vi "libdaq_adc_start_read.vi"(0 "error in (no error)":errorcluster, 1 "device_name":string, 2 "module_name":string) -> (14 "error out":errorcluster, 15 "device_name":string, 16 "module_name":string)   [LabVIEW 2022 SP3, in "libdaqVI.lvlib"]
doc: "该函数被重命名为libdaq_adc_start_task，将会在后续版本中废弃，详细功能见libdaq_adc_start_task函数；"
uses:
  libdaqVI.lvlib
  dll/daqlib.dll
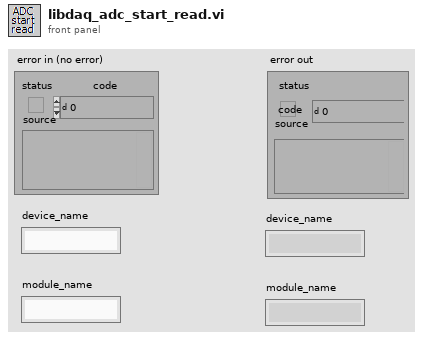
[diagram p1: front panel]
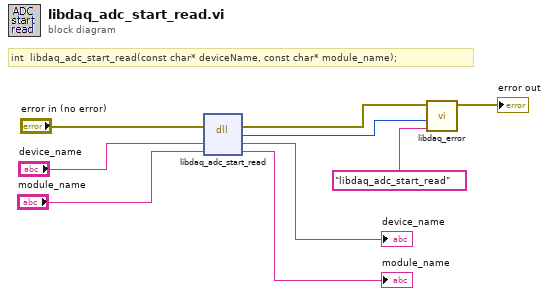
[diagram p0: block diagram]
diagram:
  # "int  libdaq_adc_start_read(const char* deviceName, const char* module_name);"
  n1 = dll-call lib="D:/Labview_projects/DAQ_USB3212/libdaqVI/dll/daqlib.dll" fn="libdaq_adc_start_read"(error in="error in (no error)", "device_name"="device_name", "module_name"="module_name") -> (error out=w3:errorcluster, "return type"=w2:i32, "device_name"=→"device_name":string, "module_name"=→"module_name":string)  [unwired: 2 in, 1 out]
  n2 = call "libdaq_error.vi"("error source"="libdaq_adc_start_read", "error code"=w2, "错误输入（无错误）"=w3) -> ("错误输出"=→"error out":errorcluster)  [unwired: 8 in]
